vi "Get Array Indices from Coords.vi"(10 "Coords":T1, 11 "Array in":refnum<vi>) -> (3 "Array Indices":cluster{i32, i32})   [LabVIEW 2019]
doc: "Converts a set of coordinates in an array to the array indices."
uses:
  <vilib>/Utility/miscctls.llb/LVPoint32TypeDef.ctl
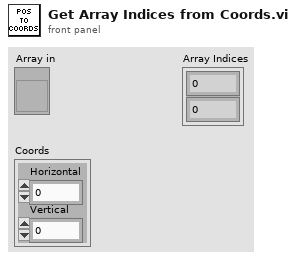
[diagram p1: front panel]
types:
  T1 = typedef "LVPoint32TypeDef.ctl" = cluster{"Horizontal":i32, "Vertical":i32}
  T2 = typedef "LVPositionTypeDef.ctl" = cluster{"Left":i32, "Top":i32}
  T3 = typedef "LVBoundsTypeDef.ctl" = cluster{"Width":u32, "Height":u32}
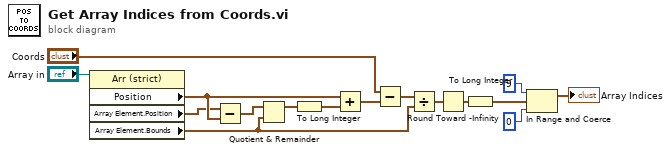
[diagram p0: block diagram]
diagram:
  n1 = property on="Property Node" class="Arr (strict)"(reference="Array in") -> ("Position"=w15:T2, "Array Element.Position"=w12:T2, "Array Element.Bounds"=w3:T3)  [unwired: 1 in, 2 out]
  n2 = Subtract(x=w12, y=w15) -> (x-y=w13:T2)
  n3 = Quotient & Remainder(x=w13, y=w3) -> (x-y*floor(x/y)=w14:T3)  [unwired: 1 out]
  n4 = To Long Integer(number=w14) -> (32bit integer=w16:cluster{"Width":i32, "Height":i32})
  n5 = Add(x=w15, y=w16) -> (x+y=w4:T2)
  n6 = Subtract(x="Coords", y=w4) -> (x-y=w10:T1)
  n7 = Divide(x=w10, y=w3) -> (x/y=w9:cluster{dbl, dbl})
  n8 = Round Toward -Infinity(1:w9) -> (0:w8:cluster{dbl, dbl})
  n9 = To Long Integer(number=w8) -> (32bit integer=w1:cluster{i32, i32})
  n10 = In Range and Coerce(upper limit=9, x=w1, lower limit=0) -> (coerced(x)=→"Array Indices":cluster{i32, i32})  [unwired: 1 out]
